vi "Run Test Test and Specific Get Method Result.vi"(8 "error in (no error)":errorcluster, 11 "Method of Interest":string) -> (0 "error out":errorcluster, 3 "Method Result out":T1)   [LabVIEW 2020, in "LUnit Tests.lvlib" / "Method Result Test.lvclass"]
uses:
  Method Result Test.lvclass
  source/Framework/Result Types/Method Result/Method Result.ctl
  source/Framework/Result Types/Assertion Result/Public/TypeDefs/Status.ctl
  source/Framework/Result Types/Assertion Result/Assertion Result.ctl
  source/Framework/Result Types/Assertion Result/Public/TypeDefs/Assertion Type.ctl
  Test Dummys/Test Test Case/Test Test Case.lvclass
  C:/Git/astemes-lunit/source/Framework/Test Case/LUnit Test Case.lvclass
  source/Framework/Execution API/Execution API.lvclass
  source/Framework/Result Types/Assertion Result/Assertion Result.lvlib
  source/Framework/Result Types/Method Result/Method Result.lvlib
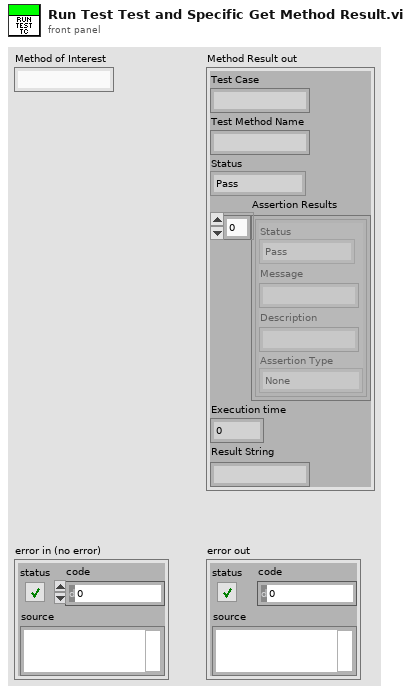
[diagram p1: front panel]
types:
  T1 = typedef "Method Result.lvlib/Method Result.ctl" = cluster{"Test Case":string, "Test Method Name":string, "Status":T2, "Assertion Results":T3[], "Execution time":dbl, "Result String":string}
  T2 = typedef "Assertion Result.lvlib/Status.ctl" = enum16{"Pass", "Fail", "Error", "Skipped", "Setup Error", "Broken", "Teardown Error"}
  T3 = typedef "Assertion Result.lvlib/Assertion Result.ctl" = cluster{"Status":T2, "Message":string, "Description":string, "Assertion Type":T4}
  T4 = typedef "Assertion Result.lvlib/Assertion Type.ctl" = enum16{"None", "Pass", "Fail", "Skip", "Pass if Equal", "Fail if Equal", "Pass if Error", "Fail if Error", "Pass if", "Fail if"}
  T5 = cluster{"Result Events":refnum<event-registration>, "Event Registration Refnum":refnum<event-registration>}
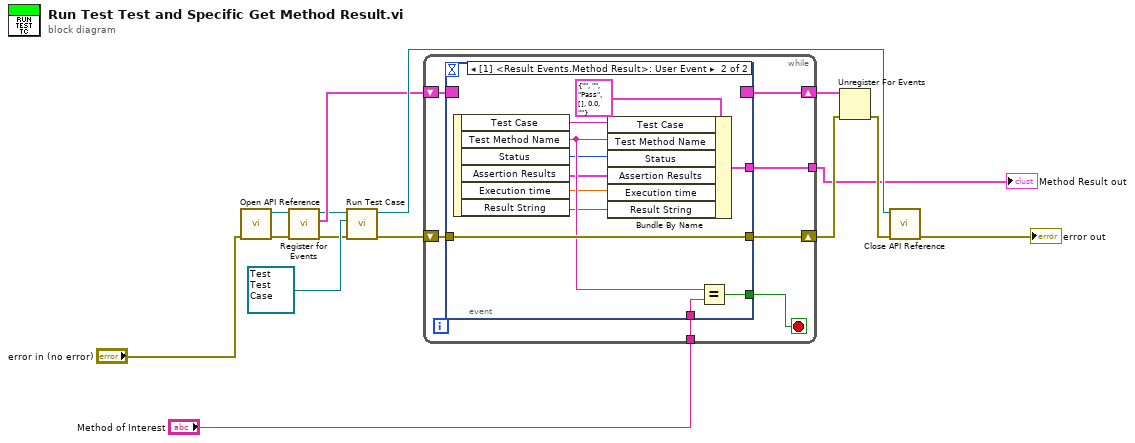
[diagram p0: block diagram]
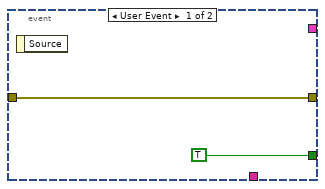
[diagram p2: hidden frame]
diagram:
  n1 = call "Open API Reference.vi"("error in (no error)"="error in (no error)") -> ("error out"=w3:errorcluster, "Execution API out"=w2:refnum<class "Execution API.lvclass">)  [unwired: 9 in]
  n2 = call "Register for Events.vi"("error in (no error)"=w3, "Execution API In"=w2) -> ("error out"=w5:errorcluster, "Result Registration Refnum"=w6:T5, "Execution API Out"=w4:refnum<class "Execution API.lvclass">)  [unwired: 7 in]
  n3 = call "Run Test Case.vi"("error in (no error)"=w5, "Test Case"=refnum<class "Test Test Case.lvclass"> refnum ("Framework Tests.lvlib:Test Test Case.lvclass"), "Execution API In"=w4) -> ("error out"=w9:errorcluster, "Execution API Out"=w13:refnum<class "Execution API.lvclass">)  [unwired: 7 in]
  n4 = while {
    shift-right: [w21] -> w7
    shift-left: w6 -> [w22]
    shift-right: [w19] -> w10
    shift-left: w9 -> [w20]
    tunnel: "Method of Interest" -> [w17]
    tunnel: [w16] -> w1
    stop <- w18 stop-if-true
    n5 = event shown="[1] <Result Events.Method Result>: User Event" {
      selector: w22 -> [_ _]
      dyn-events: [_ _] -> w21
      timeout: _ -> [_ _]
      tunnel: w20 -> [w24 w34]
      tunnel: [w24 w34] -> w19
      tunnel: [TRUE w35] -> w18
      tunnel: w17 -> [_ w33]
      tunnel: [_ w31] -> w16
      event User Event {
        n6 = event-data() -> ()  [unwired: 1 in, 1 out]
      }
      event User Event {
        n7 = event-data() -> ("Test Case"=w30:string, "Test Method Name"=w29:string, "Status"=w28:T2, "Assertion Results"=w27:T3[], "Execution time"=w26:dbl, "Result String"=w25:string)  [unwired: 1 in]
        n8 = Bundle By Name(cluster=T1 {"Test Case"="", "Test Method Name"="", "Status"=enum."Pass", "Assertion Results"=[], "Execution time"=0.0, "Result String"=""} ("Method Result out"), "Test Case"=w30, "Test Method Name"=w29, "Status"=w28, "Assertion Results"=w27, "Execution time"=w26, "Result String"=w25) -> (w31:T1)
        n9 = Equal?(x=w29, y=w33) -> (x = y?=w35:bool)
      }
    }
  }
  "Method Result out" <- w1
  n10 = Unregister For Events(event registration refnum=w7, error in=w10) -> (error out=w11:errorcluster)
  n11 = call "Close API Reference.vi"("error in (no error)"=w11, "Execution API in"=w13) -> ("error out"=→"error out":errorcluster)  [unwired: 9 in]
